vi "TwStartAcquisition.vi"(1 "error in (no error)":errorcluster) -> (0 "error out":errorcluster)   [LabVIEW 2009]
uses:
  TofDaqDll.dll
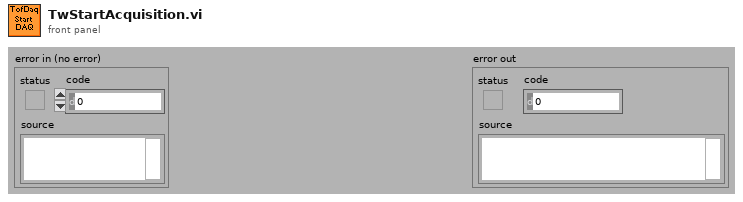
[diagram p1: front panel]
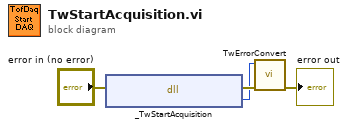
[diagram p0: block diagram]
diagram:
  n1 = dll-call lib="C:/Users/TofEmp/Desktop/LVTest/TofDaqDll.dll" fn="_TwStartAcquisition"(error in="error in (no error)") -> (error out=w3:errorcluster, "TwRetVal"=w1:i32)  [unwired: 2 in, 1 out]
  n2 = call "TwErrorConvert.vi"("error in (no error)"=w3, "error code"=w1) -> ("error out"=→"error out":errorcluster)  [unwired: 9 out]
